vi "JUnit Example.vi"() -> ()   [LabVIEW 2013]
uses:
  Controls/Test Suite Attribute Values.ctl
  Controls/Test Case Attributes.ctl
  Controls/Outcome Attributes.ctl
  <vilib>/xml/Close Reference(Node).vi
  <vilib>/xml/NI_XML.lvlib
  JUnit API.lvlib
panel:
  out "Error Out":errorcluster
  in  "Error In (No Error)":errorcluster
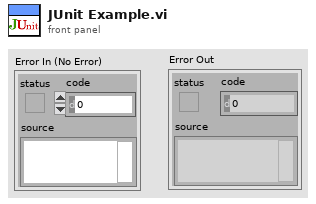
[diagram p1: front panel]
types:
  T1 = typedef "JUnit API.lvlib/Test Suite Attribute Values.ctl" = cluster{"name":string, "tests":i32, "failures":i32, "errors":i32, "time":dbl, "disabled":i32, "skipped":i32, "skips":i32, "timestamp":dbl, "hostname":string, "id":string, "package":string, "assertions":i32, "file":string, "skip":string, "log":string, "url":string}
  T2 = typedef "JUnit API.lvlib/Outcome Attributes.ctl" = cluster{"message":string, "type":string}
  T3 = typedef "JUnit API.lvlib/Test Case Attributes.ctl" = cluster{"name":string, "assertions":i32, "time":dbl, "timestamp":dbl, "classname":string, "status":string, "class":string, "file":string, "line":string, "log":string, "group":string, "url":string}
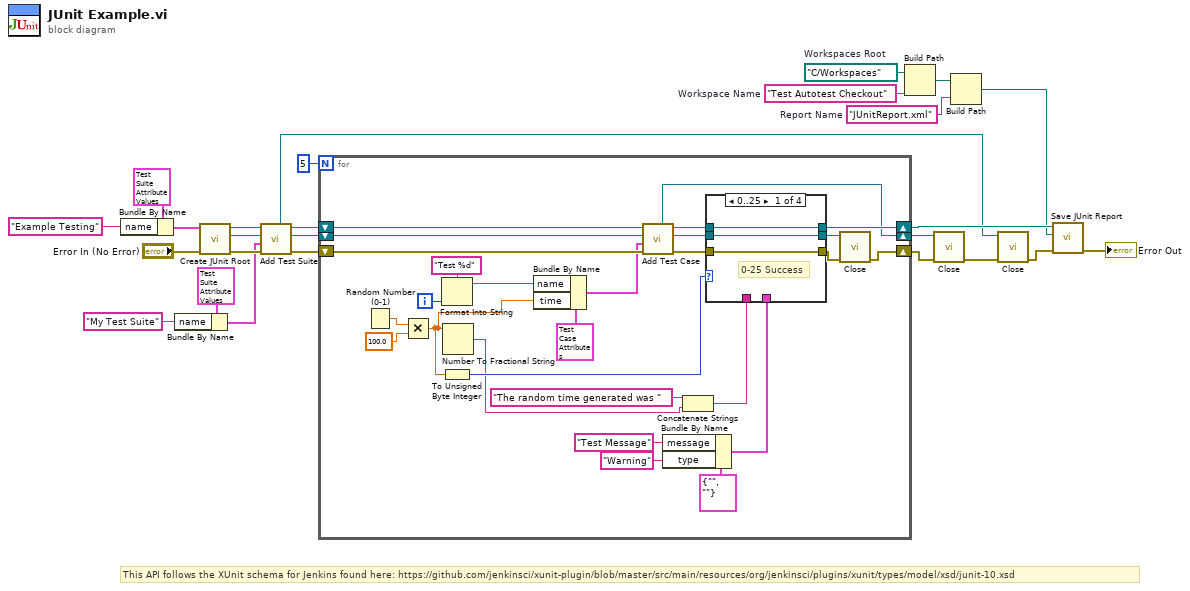
[diagram p0: block diagram]
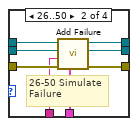
[diagram p2: hidden frame]
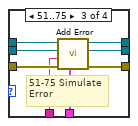
[diagram p3: hidden frame]
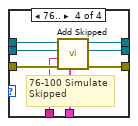
[diagram p4: hidden frame]
diagram:
  w24 = "Test Autotest Checkout"  # Workspace Name
  w23 = path "C:/Workspaces"  # Workspaces Root
  w22 = "JUnitReport.xml"  # Report Name
  # "This API follows the XUnit schema for Jenkins found here: https://github.com/jenkinsci/xunit-plugin/blob/master/src/main/resources/org/jenkinsci/plugins/xunit/types/model/xsd/junit-10.xsd"
  n1 = Bundle By Name(cluster=T1 {"name"="", "tests"=-1, "failures"=-1, "errors"=-1, "time"=-1.0, "disabled"=-1, "skipped"=-1, "skips"=-1, "timestamp"=-1.0, "hostname"="", "id"="", "package"="", "assertions"=-1, "file"="", "skip"="", "log"="", "url"=""} ("Test Suites Atrributes"), "name"="Example Testing" ("name.Attribute Value")) -> (w2:T1)
  n2 = Bundle By Name(cluster=T1 {"name"="", "tests"=-1, "failures"=-1, "errors"=-1, "time"=-1.0, "disabled"=-1, "skipped"=-1, "skips"=-1, "timestamp"=-1.0, "hostname"="", "id"="", "package"="", "assertions"=-1, "file"="", "skip"="", "log"="", "url"=""} ("Test Suites Atrributes"), "name"="My Test Suite" ("name.Attribute Value")) -> (w5:T1)
  n3 = call "Create JUnit Root.vi"("Error In (No Error)"="Error In (No Error)", "Test Suites Atrributes"=w2) -> ("Error Out"=w20:errorcluster, "Teststuites Ref"=w17:refnum<k20>, "File Ref Out"=w18:refnum<k20>)  [unwired: 7 in]
  n4 = call "Add Test Suite.vi"("Error In (No Error)"=w20, "Test Suite Atrributes"=w5, "Teststuites Ref In"=w17, "File Ref In"=w18) -> ("Error Out"=w19:errorcluster, "Testsuite Ref"=w16:refnum<k20>, "File Ref Out"=w15:refnum<k20>, "Teststuites Ref Out"=w9:refnum<k20>)  [unwired: 4 in]
  n5 = for {
    N: 5 -> [_]
    shift-right: [w38] -> w13
    shift-left: w19 -> [w53]
    shift-right: [w46] -> w12
    shift-left: w16 -> [w51]
    shift-right: [w47] -> w14
    shift-left: w15 -> [w50]
    i -> [w43]
    n6 = Random Number (0-1)() -> (number: 0 to 1=w42:dbl)
    n7 = Multiply(x=w42, y=100.0) -> (x*y=w27:dbl)
    n8 = Format Into String(format string="Test %d", w43) -> (resulting string=w44:string)  [unwired: 2 in, 1 out]
    n9 = To Unsigned Byte Integer(number=w27) -> (unsigned 8bit integer=w31:u8)
    n10 = Number To Fractional String(number=w27) -> (F-format string=w29:string)  [unwired: 3 in]
    n11 = Bundle By Name(cluster=T3 {"name"="", "assertions"=-1, "time"=-1.0, "timestamp"=-1.0, "classname"="", "status"="", "class"="", "file"="", "line"="", "log"="", "group"="", "url"=""} ("Test Case Atrributes"), "name"=w44, "time"=w27) -> (w36:T3)
    n12 = call "Add Test Case.vi"("Error In (No Error)"=w53, "Test Case Atrributes"=w36, "Testsuite Ref In"=w51, "File Ref In"=w50) -> ("error out"=w52:errorcluster, "Testcase Ref"=w49:refnum<k20>, "File Ref Out"=w48:refnum<k20>, "Testsuite Ref Out"=w46:refnum<k20>)  [unwired: 4 in]
    n13 = Bundle By Name(cluster=T2 {"message"="", "type"=""} ("Failure Attributes"), "message"="Test Message", "type"="Warning") -> (w32:T2)
    n14 = Concatenate Strings("The random time generated was " ("Text"), w29) -> (w28:string)
    n15 = case shown="0..25" w31 {
      tunnel: w52 -> [w55 w64 w72 w80]
      tunnel: w49 -> [w54 w63 w71 w79]
      tunnel: w48 -> [w56 w62 w70 w78]
      tunnel: [w55 w61 w69 w77] -> w39
      tunnel: [w56 w60 w68 w76] -> w47
      tunnel: [w54 w59 w67 w75] -> w40
      tunnel: w28 -> [_ w58 w66 w74]
      tunnel: w32 -> [_ w57 w65 w73]
      frame 0..25 {
        # "0-25 Success"
      }
      frame 26..50 {
        # "26-50 Simulate\nFailure"
        n16 = call "Add Failure.vi"("Outcome Attributes"=w57, "Error In (No Error)"=w64, "Text"=w58, "Testcase Ref"=w63, "File Ref In"=w62) -> ("Error Out"=w61:errorcluster, "Testcase Ref Out"=w59:refnum<k20>, "File Ref Out"=w60:refnum<k20>)  [unwired: 4 in]
      }
      frame 51..75 {
        # "51-75 Simulate\nError"
        n17 = call "Add Error.vi"("Outcome Attributes"=w65, "Error In (No Error)"=w72, "Text"=w66, "Testcase Ref"=w71, "File Ref In"=w70) -> ("Error Out"=w69:errorcluster, "Testcase Ref Out"=w67:refnum<k20>, "File Ref Out"=w68:refnum<k20>)  [unwired: 4 in]
      }
      frame 76.. {
        # "76-100 Simulate\nSkipped"
        n18 = call "Add Skipped.vi"("Outcome Attributes"=w73, "Error In (No Error)"=w80, "Text"=w74, "Testcase Ref"=w79, "File Ref In"=w78) -> ("Error Out"=w77:errorcluster, "Testcase Ref Out"=w75:refnum<k20>, "File Ref Out"=w76:refnum<k20>)  [unwired: 4 in]
      }
    }
    n19 = call-poly <vilib>:"Close.vi"("error in (no error)"=w39, "node"=w40) -> ("error out"=w38:errorcluster)  [unwired: 7 in]
  }
  n20 = Build Path(base path=w23, name or relative path=w24) -> (appended path=w25:path)
  n21 = call-poly <vilib>:"Close.vi"("error in (no error)"=w13, "node"=w12) -> ("error out"=w10:errorcluster)  [unwired: 7 in]
  n22 = Build Path(base path=w25, name or relative path=w22) -> (appended path=w1:path)
  n23 = call-poly <vilib>:"Close.vi"("error in (no error)"=w10, "node"=w9) -> ("error out"=w8:errorcluster)  [unwired: 7 in]
  n24 = call "Save JUnit Report.vi"("Error In (No Error)"=w8, "XML file path"=w1, "File Ref In"=w14) -> ("Error Out"=→"Error Out":errorcluster)  [unwired: 8 in]
